vi "读TDMS文件.vi"() -> ()   [LabVIEW 2010]
doc: "Reads Channel groups from a storage."
panel:
  in  "文件路径":path=path "F:/c7/prog7/TDMSFile.tdms"
  out "属性值":variant[](array[variant])=[variant(u64 100), variant(u16 10), variant(string "YD68"), variant(timestamp timestamp(0 s since 1904-01-01)), variant(dbl 0.0), variant(dbl 0.001), variant(i32 100), variant(string "正弦"), variant(bool TRUE), variant(string "relative"), variant(timestamp timestamp(3275473672.484375 s since 1904-01-01)), variant(timestamp timestamp(3275473672.484375 s since 1904-01-01)), variant(string "t"), variant(string "Time"), variant(string "s")]
  out "通道属性":string[](array[string])=["NI_ChannelLength", "NI_DataType", "传感器", "wf_start_time", "wf_start_offset", "wf_increment", "wf_samples", "NI_ChannelName", "NI_ExpIsRelativeTime", "wf_time_pref", "NI_ExpStartTimeStamp", "NI_ExpTimeStamp", "NI_ExpXDimension", "wf_xname", "wf_xunit_string"]
  out "组属性":string[](array[string])=["采样率"]
  out "属性值":variant[](array[variant])=[variant(dbl 1024.0)]
  out "?":variant[](array[variant])=[variant(string "示例程序"), variant(string "赵晨光")]
  out "?":string[](array[string])=["测试系统", "操作人员"]
  out "波形图":dbl[][](graph)=[[0.0, 0.0634175857813252, 0.1265798623799041, 0.18923254844743084, 0.2511234141665813, 0.3120032966884148, 0.3716271032226454, 0.4297547977425003, 0.4861523673318466, 0.5405927642842268, 0.5928568201610591, 0.6427341281291522, 0.6900238900253773, 0.7345357247383564, 0.7760904346527414, 0.8145207270705094, 0.8496718877049362, 0.8814024035358785, 0.9095845325188363, 0.9341048178542484, 0.9548645447466428, 0.9717801378148127, 0.9847834975530967, 0.993822274489234, 0.9988600799350685, 0.9998766324816606, 0.9968678396490348, 0.9898458143618585, 0.9788388261847202, 0.9638911875133281, 0.9450630751798048, 0.9224302881902667, 0.8960839425699989, 0.8661301045447303, 0.8326893635347631, 0.7958963466810159, 0.7558991768574196, 0.7128588763516256, 0.6669487186147105, 0.6183535306896335, 0.5672689491267566, 0.5139006323819968, 0.458463432868368, 0.40118053199410575, 0.3422825416695715, 0.28200657590012973, 0.22059529620261753, 0.15829593468840908, 0.09535929874598903, 0.03203876133002422, -0.03141075907812785, -0.09473382473195789, -0.15767550697182214, -0.21998241252745737, -0.2814037036392598, -0.3416921078914828, -0.40060491369192236, -0.45790494739044835, -0.5133615281026551, -0.5667513963946633, -0.6178596130903338, -0.6664804245824388, -0.7124180911641828, -0.7554876750463428, -0.7955157848875944, -0.832341273840663, -0.8658158883040745, -0.8958048647677382, -0.9221874723495489, -0.944857498838849, -0.9637236782900093, -0.9787100584447116, -0.9897563065037406, -0.9968179520173057, -0.9998665659160451, -0.9988898749619699, -0.99389181115858, -0.9848924959212413, -0.9719281590715428, -0.9550509929817614, -0.934328942456612, -0.9098454311981998, -0.8816990259553703, -0.8500030397095515, -0.8148850754945864, -0.776486512687079, -0.7349619378353532, -0.6904785223184312, -0.6432153493404656, -0.593362692970051, -0.5411212521268765, -0.48670134259958137, -0.43032205034760956, -0.3722103494957459, -0.312600188572142, -0.251731548668498, -0.18984947731409485, -0.1272031019531499, -0.06404462699707955, -0.0006283184893772641], [0.0, 0.0202, 0.0404, 0.0606, 0.0808, 0.101, 0.1212, 0.1414, 0.1616, 0.1818, 0.202, 0.22219999999999998, 0.2424, 0.2626, 0.2828, 0.303, 0.3232, 0.3434, 0.3636, 0.38380000000000003, 0.404, 0.42419999999999997, 0.44439999999999996, 0.4646, 0.4848, 0.505, 0.5252, 0.5454, 0.5656, 0.5858, 0.606, 0.6262, 0.6464, 0.6666, 0.6868, 0.707, 0.7272, 0.7474, 0.7676000000000001, 0.7878000000000001, 0.808, 0.8282, 0.8483999999999999, 0.8685999999999999, 0.8887999999999999, 0.909, 0.9292, 0.9494, 0.9696, 0.9898, -0.9900000000000001, -0.9698000000000001, -0.9496, -0.9294, -0.9092, -0.889, -0.8688, -0.8486, -0.8283999999999999, -0.8081999999999999, -0.7879999999999999, -0.7678, -0.7476, -0.7274, -0.7072, -0.6869999999999999, -0.6668, -0.6466, -0.6264, -0.6062000000000001, -0.5860000000000001, -0.5657999999999999, -0.5456000000000001, -0.5254, -0.5052000000000001, -0.485, -0.4647999999999999, -0.44460000000000005, -0.42439999999999994, -0.4042000000000001, -0.38399999999999995, -0.3638000000000001, -0.3436, -0.32339999999999985, -0.3032000000000001, -0.2829999999999999, -0.2628000000000001, -0.24259999999999995, -0.22240000000000015, -0.20220000000000002, -0.18199999999999988, -0.16180000000000005, -0.14159999999999992, -0.1214000000000001, -0.10119999999999997, -0.08100000000000016, -0.06080000000000002, -0.040599999999999886, -0.020400000000000067, -0.00019999999999993124], [-0.09693384783092193, 0.6029566069934109, -0.19511619830427984, 0.20062612811282682, -0.19451360223997938, -0.1386448755328597, 0.11353813641623728, 0.4815649598474745, 0.658078457569508, 0.290046170688353, 0.8448978318407798, 0.11628845271738308, 0.4919227221729049, 0.3162141577704007, 1.372887071259926, 0.812383792764611, 0.5911656762353368, 1.178768488064403, 1.3832615660044931, 0.5851595287378616, 0.36648580201631886, 1.0266466074721667, 0.4879587220470882, 1.077459827842705, 0.5108274439057907, 0.4351580117965247, 1.2073826777222687, 1.3293496573009687, 1.0695142862914635, 0.5352516096770288, 0.8150974299717224, 1.0986533740307285, 0.3100913107364768, 1.385707656771356, 0.6997490980867532, 0.4166308630182135, 0.522906905729465, 0.8697309883177851, 0.3014166846686626, 0.8896836024782993, 0.5953928677980623, 0.5339018667101316, 0.04484915914973775, 0.3870936566930653, 0.3587247046093676, 0.5325472225692817, 0.6685494181047111, 0.3045388573870174, 0.14146877396205532, -0.5077900755221005, -0.11577901866044357, -0.48996530859564347, -0.536373747620782, -0.268594337523059, -0.6808328008651077, -0.4647089473504293, -0.35843171853168737, -1.0031579417077994, -0.8631417702584896, -0.058119134787734006, -0.2488135435201187, -1.187088277651906, -1.1902364439555189, -0.40452183981687634, -1.2581602096978834, -0.47061999407464883, -0.7937854184535291, -1.088105905177663, -0.5618161702709461, -1.0120411729706096, -1.2144006868596768, -0.7645081711972249, -0.6736481688112312, -1.3212251203044212, -0.6544856373037574, -0.8400689597425148, -1.4423043402922961, -1.0505462402310501, -1.2794844390550413, -0.43583402574761754, -0.4717308557763381, -0.4499953691224049, -0.6031275401642903, -1.1726514054245039, -0.47699179519884644, -0.3054816422221445, -0.9183068829171649, -0.31847236326788986, -0.8262637988462072, -0.48070838337574107, -0.09787381935253253, -0.13158124996063414, 0.04913157452173861, -0.16349823483790413, -0.006167716598680317, 0.0064962942590013895, 0.33350128265813905, -0.09393433483791566, 0.37121783256808416, -0.3798838756812302], [1.0, 1.0202, 0.0404, 0.0606, 1.0808, 0.101, 1.1212, 1.1414, 1.1616, 0.1818, 0.202, 1.2222, 0.2424, 1.2626, 1.2828, 1.303, 0.3232, 0.3434, 1.3636, 0.38380000000000003, 1.404, 1.4242, 1.4444, 0.4646, 0.4848, 1.505, 0.5252, 1.5453999999999999, 1.5655999999999999, 1.5857999999999999, 0.606, 0.6262, 1.6463999999999999, 0.6666, 1.6867999999999999, 1.7069999999999999, 1.7271999999999998, 0.7474, 0.7676000000000001, 1.7878, 0.808, 1.8282, 1.8483999999999998, 1.8685999999999998, 0.8887999999999999, 0.909, 1.9292, 0.9494, 1.9696, 1.9898, 0.009999999999999898, -0.9698000000000001, -0.9496, 0.0706, -0.9092, 0.11099999999999999, 0.13119999999999998, 0.15139999999999998, -0.8283999999999999, -0.8081999999999999, 0.21200000000000008, -0.7678, 0.25239999999999996, 0.27259999999999995, 0.29279999999999995, -0.6869999999999999, -0.6668, 0.35340000000000005, -0.6264, 0.39379999999999993, 0.4139999999999999, 0.43420000000000014, -0.5456000000000001, -0.5254, 0.4947999999999999, -0.485, 0.5352000000000001, 0.5553999999999999, 0.5756000000000001, -0.4042000000000001, -0.38399999999999995, 0.6361999999999999, -0.3436, 0.6766000000000001, 0.6967999999999999, 0.7170000000000001, -0.2628000000000001, -0.24259999999999995, 0.7775999999999998, -0.20220000000000002, 0.8180000000000001, 0.8382, 0.8584, -0.1214000000000001, -0.10119999999999997, 0.9189999999999998, -0.06080000000000002, 0.9594000000000001, 0.9795999999999999, 0.9998]]
  # "读取TDMS文件数据面板"
  # "文件属性"
  # "属性值"
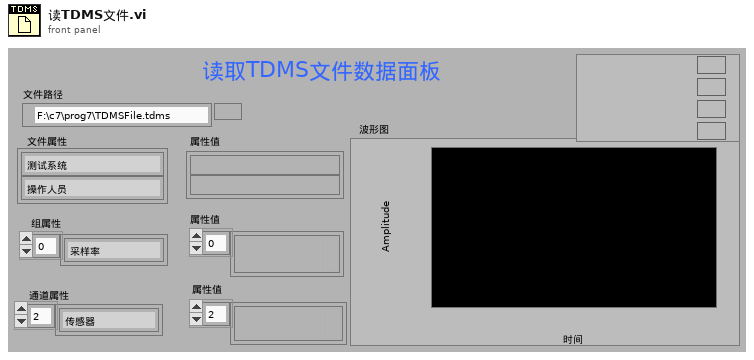
[diagram p1: front panel]
types:
  T1 = enum16{"open", "open or create", "create or replace", "create", "open (read-only)"}
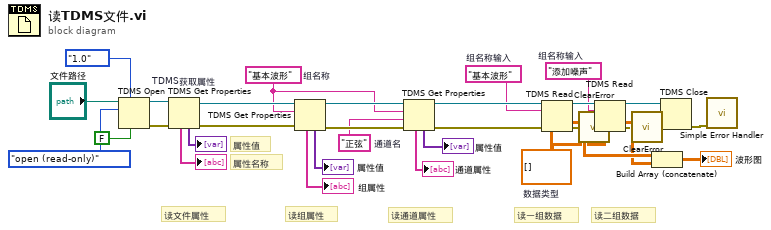
[diagram p0: block diagram]
diagram:
  w5 = "添加噪声"  # 组名称输入
  w7 = dbl[][] []  # 数据类型
  w14 = "基本波形"  # 组名称输入
  w20 = "正弦"  # 通道名
  w21 = "基本波形"  # 组名称
  # "读二组数据"
  # "读一组数据"
  # "读通道属性"
  # "读组属性"
  # "读文件属性"
  # "属性名称"
  # "属性值"
  n1 = TDMS Open(6:FALSE ("禁用缓冲？(T)"), 7:enum16{"1.0", "2.0"}."1.0" ("文件格式版本(2.0)"), 10:T1."open (read-only)" ("operation"), 11:"文件路径") -> (0:w29:errorcluster, 3:w28:refnum<k34>)  [unwired: 2 in]
  n2 = TDMS Get Properties "TDMS获取属性"(8:w29, 11:w28) -> (0:w26:errorcluster, 3:w27:refnum<k34>, 4:→"?":variant[], 6:→"?":string[])  [unwired: 4 in, 2 out]
  n3 = TDMS Get Properties(8:w26, 10:w21, 11:w27) -> (0:w22:errorcluster, 3:w23:refnum<k34>, 4:→"属性值":variant[], 6:→"组属性":string[])  [unwired: 3 in, 2 out]
  n4 = TDMS Get Properties(8:w22, 9:w20, 10:w21, 11:w23) -> (0:w15:errorcluster, 3:w16:refnum<k34>, 4:→"属性值":variant[], 6:→"通道属性":string[])  [unwired: 2 in, 2 out]
  n5 = TDMS Read(0:w16, 5:w14, 11:w15, 12:w7) -> (4:w13:refnum<k34>, 10:w9:dbl[][], 15:w3:errorcluster)  [unwired: 3 in, 3 out]
  n6 = call <vilib>:"ClearError.vi"("error in (no error)"=w3) -> ("error out"=w12:errorcluster)
  n7 = TDMS Read(0:w13, 5:w5, 11:w12, 12:w7) -> (4:w11:refnum<k34>, 10:w8:dbl[][], 15:w4:errorcluster)  [unwired: 3 in, 3 out]
  n8 = call <vilib>:"ClearError.vi"("error in (no error)"=w4) -> ("error out"=w10:errorcluster)
  n9 = Build Array (concatenate)(w9, w8) -> (→"波形图":dbl[][])
  n10 = TDMS Close(8:w10, 11:w11) -> (0:w33:errorcluster)  [unwired: 1 out]
  n11 = call <vilib>:"Simple Error Handler.vi"("error in (no error)"=w33) -> ()  [unwired: 4 in, 5 out]
